vi "Write Device.vi"(8 "error in (no error)":errorcluster, 10 "Device":i32, 11 "ATS660 Class in":refnum<class "ATS660 Class.lvclass">) -> (0 "error out":errorcluster, 3 "ATS660 Class out":refnum<class "ATS660 Class.lvclass">)   [LabVIEW 2015, in "ATS660 Class.lvclass"]
uses:
  ATS660 Class.lvclass
  ATS660 Class.lvclass/ATS660 Class.ctl
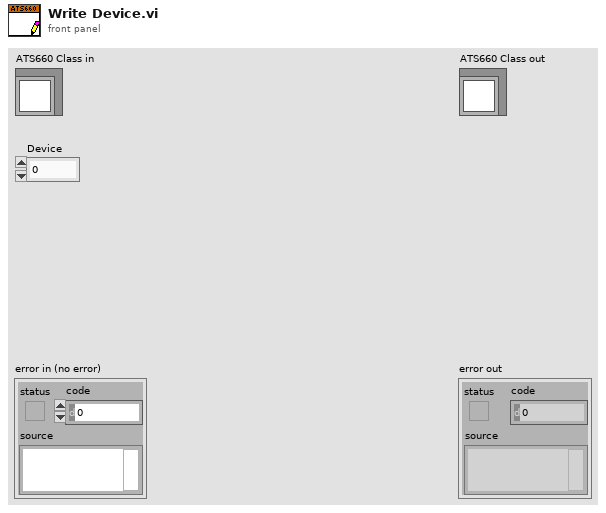
[diagram p1: front panel]
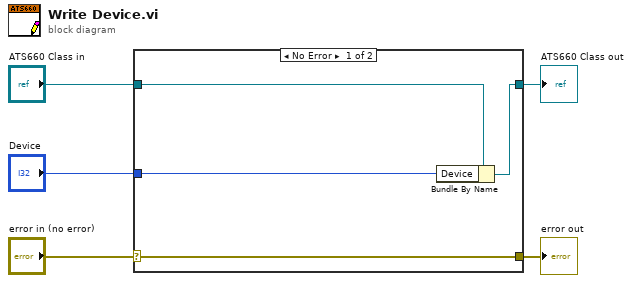
[diagram p0: block diagram]
diagram:
  n1 = case shown="No Error" "error in (no error)" {
    selector: "error in (no error)" -> [w9 w10]
    tunnel: [w9 w10] -> w4
    tunnel: [w7 w11] -> w2
    tunnel: "ATS660 Class in" -> [w8 w11]
    tunnel: "Device" -> [w6 _]
    frame No Error {
      n2 = Bundle By Name(cluster=w8, "Device"=w6) -> (w7:refnum<class "ATS660 Class.lvclass">)
    }
    frame Error {
    }
  }
  "error out" <- w4
  "ATS660 Class out" <- w2
